vi "fakespectra_2.vi"(0 "all rows":dbl[][](array[numeric]) format="%0.3f", 1 "LT preset":dbl) -> (2 "Waveform Graph":u32[](graph), 3 "LT out":dbl, 4 "RT out":dbl)   [LabVIEW 2015]
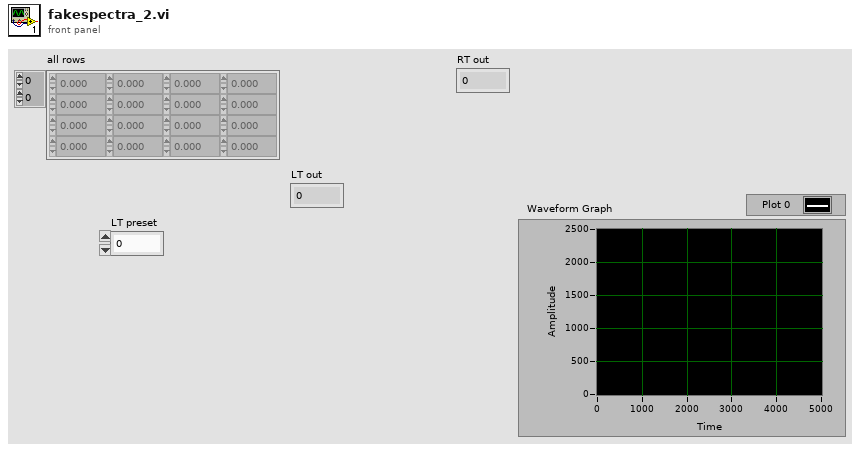
[diagram p1: front panel]
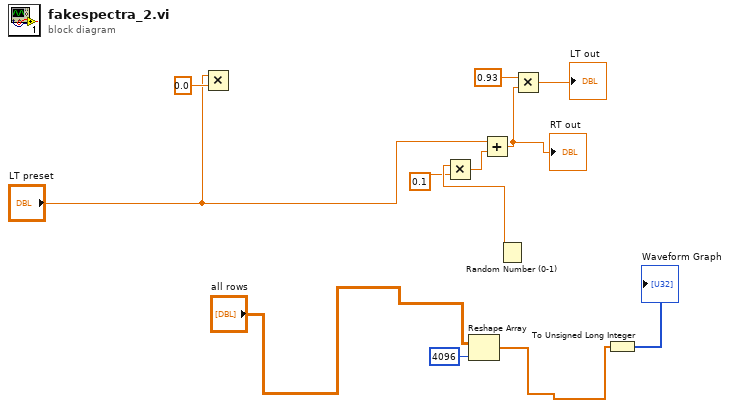
[diagram p0: block diagram]
diagram:
  n1 = Multiply(x="LT preset", y=0.0) -> ()  [unwired: 1 out]
  n2 = Reshape Array("all rows", 4096 ("dimension size")) -> (w2:dbl[])
  n3 = Random Number (0-1)() -> (number: 0 to 1=w10:dbl)
  n4 = Multiply(x=w10, y=0.1) -> (x*y=w8:dbl)
  n5 = Add(x="LT preset", y=w8) -> (x+y=w4:dbl)
  "RT out" <- w4
  n6 = Multiply(x=0.93, y=w4) -> (x*y=→"LT out":dbl)
  n7 = To Unsigned Long Integer(number=w2) -> (unsigned 32bit integer=→"Waveform Graph":u32[])
